vi "Create Message - Value Change & Trigger.vi"(7 "optional settings":T2, 8 "error in (no error)":errorcluster, 10 "message name":string, 11 "message group refnum in":u64 format="%.0x") -> (0 "error out":errorcluster, 2 "message refnum out":T1 format="%.0x", 3 "message group refnum out":T1 format="%.0x")   [LabVIEW 2018, in "Instrument Addon Scripting API.lvlib"]
doc: "Creates a new message section which has \"Value Change & Trigger\" setting set as the \"Generation Type\".\n\"Value Change & Trigger\" will trigger the message by using the Trigger Channel or anytime a VeriStand channel used in the command field is changed. If the command message contains multiple VeriStand channels, the message will be sent each time one of the channel has changed."
uses:
  Instrument Addon Scripting API.lvlib
  <vilib>/NI Veristand/Custom Device API/Custom Device Channel Type.ctl
  <vilib>/NI Veristand/Custom Device API/Custom Device API.lvlib
  <vilib>/NI Veristand/Custom Device API/Custom Device Channel.ctl
  Addon/Addon Shared/Types/Message Generation Type.ctl
  Addon/Addon Shared/Instrument Addon Shared.lvlib
  TypeDefs/Protection Types.ctl
  TypeDefs/Message Settings.ctl
  <vilib>/NI Veristand/Custom Device API/Custom Device Item Ref.ctl
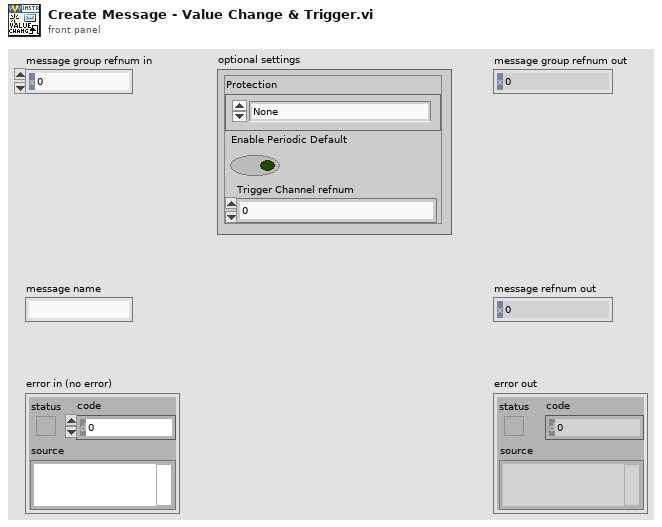
[diagram p1: front panel]
types:
  T1 = typedef "Custom Device API.lvlib/Custom Device Item Ref.ctl" = u64
  T2 = typedef "Instrument Addon Scripting API.lvlib/Message Settings.ctl" = cluster{"Protection":T3, "Enable Periodic Default":bool, "Trigger Channel refnum":u64}
  T3 = typedef "Instrument Addon Scripting API.lvlib/Protection Types.ctl" = enum16{"None", "CRC-32", "Checksum U16", "Checksum U32", "Checksum U8"}
  T4 = typedef "Instrument Addon Shared.lvlib/Message Generation Type.ctl" = enum16{"Trigger Only", "Periodic & Trigger", "Value Change & Trigger"}
  T5 = typedef "Custom Device API.lvlib/Custom Device Channel.ctl" = cluster{"Type":T6, "Units":string, "Default Value":dbl, "Faultable":bool, "Scalable":bool}
  T6 = typedef "Custom Device API.lvlib/Custom Device Channel Type.ctl" = enum16{"Input", "Output"}
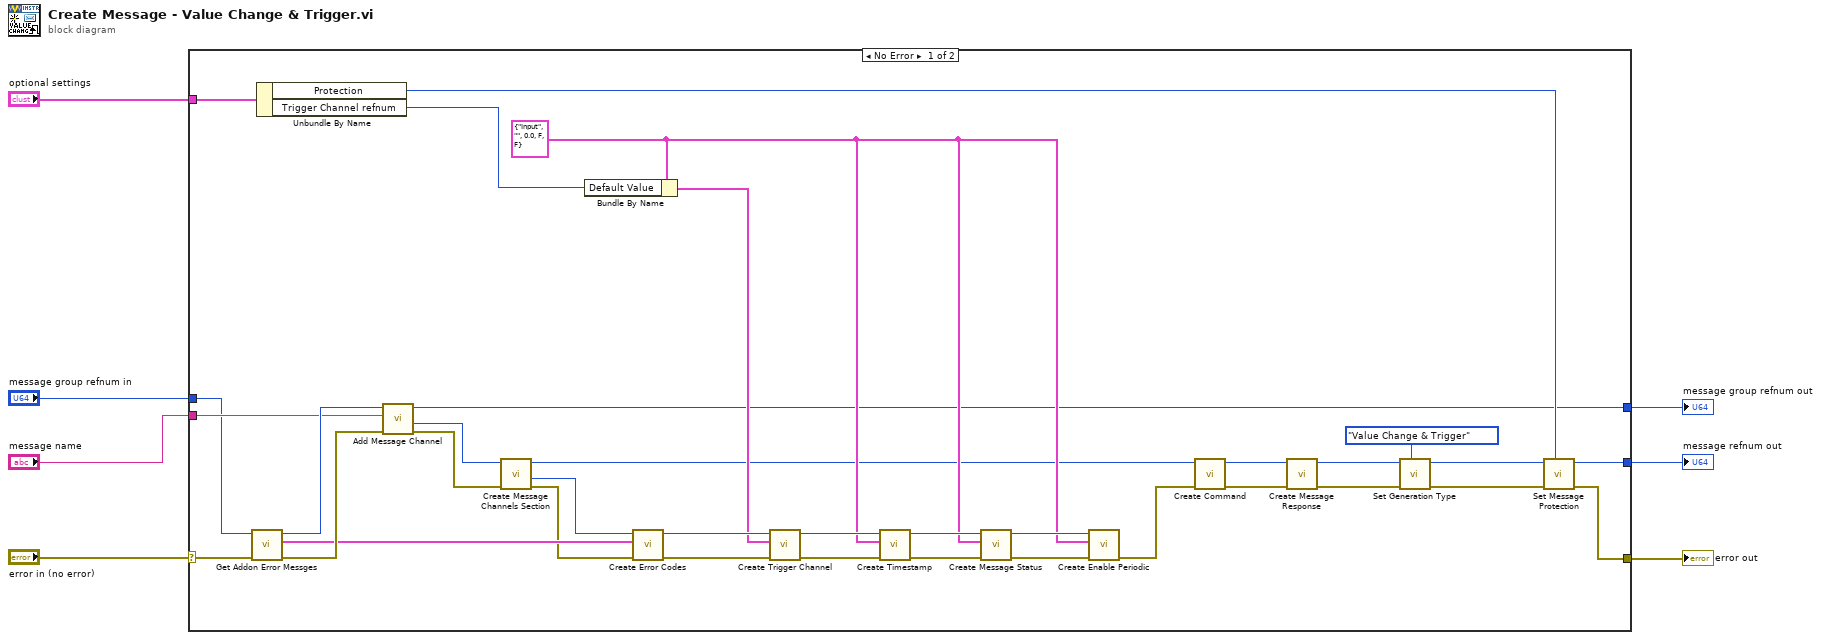
[diagram p0: block diagram]
diagram:
  n1 = case shown="No Error" "error in (no error)" {
    selector: "error in (no error)" -> [w9 w43]
    tunnel: [w21 w43] -> w7
    tunnel: "optional settings" -> [w17 _]
    tunnel: "message name" -> [w16 _]
    tunnel: [w15 _] -> w4
    tunnel: [w14 _] -> w3
    tunnel: "message group refnum in" -> [w8 _]
    frame No Error {
      w20 = T5 {"Type"=enum."Input", "Units"="", "Default Value"=0.0, "Faultable"=FALSE, "Scalable"=FALSE} ("Channel")
      n2 = call "Get Addon Error Messges.vi"("error in (no error)"=w9, "Message Group in"=w8) -> ("error out"=w38:errorcluster, "Error Messages out"=w35:cluster{"Code":i32, "String":string}[], "Message Group out"=w34:u64)  [unwired: 7 in]
      n3 = Unbundle By Name(w17) -> ("Protection"=w22:T3, "Trigger Channel refnum"=w18:u64)
      n4 = call "Add Message Channel.vi"("error in (no error)"=w38, "Message Name"=w16, "Message Goup in"=w34) -> ("error out"=w42:errorcluster, "Message out"=w36:T1, "Message Goup out"=w15:T1)  [unwired: 6 in]
      n5 = call "Create Message Channels Section.vi"("error in (no error)"=w42, "Message in"=w36) -> ("error out"=w33:errorcluster, "Message Channels Section out"=w32:T1, "Message out"=w10:T1)  [unwired: 7 in]
      n6 = Bundle By Name(cluster=w20, "Default Value"=w18) -> (w19:T5)
      n7 = call "Create Error Codes.vi"("error in (no error)"=w33, "Error Codes"=w35, "Message Channels Section in"=w32) -> ("error out"=w30:errorcluster, "Message Channels Section out"=w31:T1)  [unwired: 7 in]
      n8 = call "Create Trigger Channel.vi"("error in (no error)"=w30, "Channel Parameters"=w19, "Message Channels Section in"=w31) -> ("error out"=w29:errorcluster, "Message Channels Section out"=w28:T1)  [unwired: 6 in, 1 out]
      n9 = call "Create Timestamp.vi"("error in (no error)"=w29, "Channel Paramters"=w20, "Message Channels Section in"=w28) -> ("error out"=w41:errorcluster, "Message Channels Section out"=w37:T1)  [unwired: 6 in, 1 out]
      n10 = call "Create Message Status.vi"("error in (no error)"=w41, "Channel Paramters"=w20, "Message Channels Section in"=w37) -> ("error out"=w40:errorcluster, "Message Channels Section out"=w39:T1)  [unwired: 7 in]
      n11 = call "Create Enable Periodic.vi"("error in (no error)"=w40, "Channel Parameters"=w20, "Message Channels Section in"=w39) -> ("error out"=w11:errorcluster)  [unwired: 7 in, 1 out]
      n12 = call "Create Command.vi"("error in"=w11, "message refnum In"=w10) -> ("error out"=w13:errorcluster, "message refnum out"=w12:T1)  [unwired: 7 in, 1 out]
      n13 = call "Create Message Response.vi"("Error In"=w13, "Message Refnum In"=w12) -> ("Error Out"=w27:errorcluster, "Message Refnum Out"=w25:T1)  [unwired: 7 in, 1 out]
      n14 = call "Set Generation Type.vi"("Generation Type"=Message_Generation_Type."Value Change & Trigger", "error in (no error)"=w27, "Message in"=w25) -> ("error out"=w24:errorcluster, "Message out"=w23:T1)  [unwired: 7 in]
      n15 = call "Set Message Protection.vi"("Protection Type"=w22, "error in (no error)"=w24, "Message in"=w23) -> ("error out"=w21:errorcluster, "Message out"=w14:T1)  [unwired: 7 in]
    }
    frame Error {
    }
  }
  "error out" <- w7
  "message group refnum out" <- w4
  "message refnum out" <- w3
